vi "eventp.vi"() -> ()   [LabVIEW 2020]
panel:
  out "error out 2":errorcluster
  out "refnum out 2":refnum<file>
  in  "Write":bool
  out "refnum out":refnum<file>
  out "error out":errorcluster
  in  "Close File":bool
  in  "Path":path=path "C:/Users/rsKite/Documents/FSR DATA"
  out "File Name":string
  in  "Weight":string
  in  "Trial":string caption="Participant Name (FirstLast)"
  in  "Create/OpenFile":bool
  in  "OK Button":bool
  in  "stop":bool
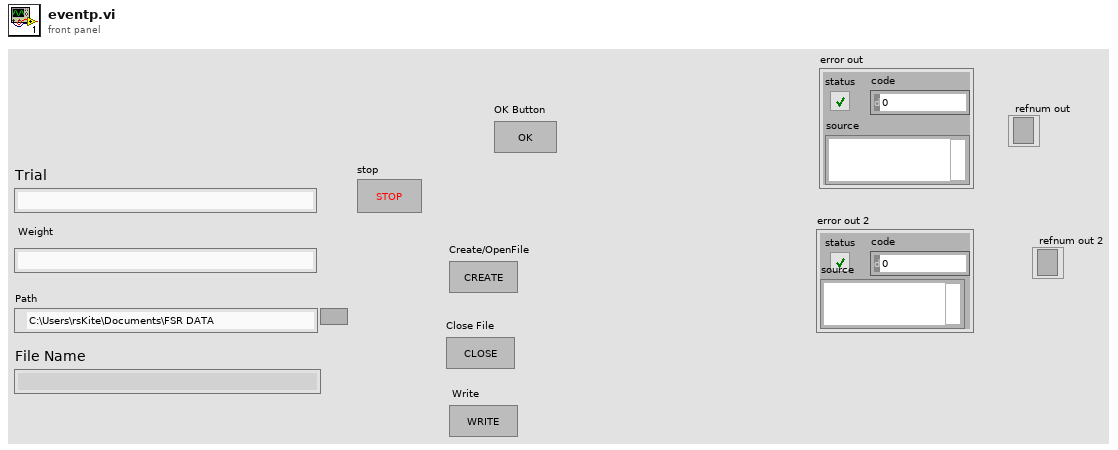
[diagram p1: front panel]
types:
  T1 = enum16{"open", "replace", "create", "open or create", "replace or create", "replace or create with confirmation"}
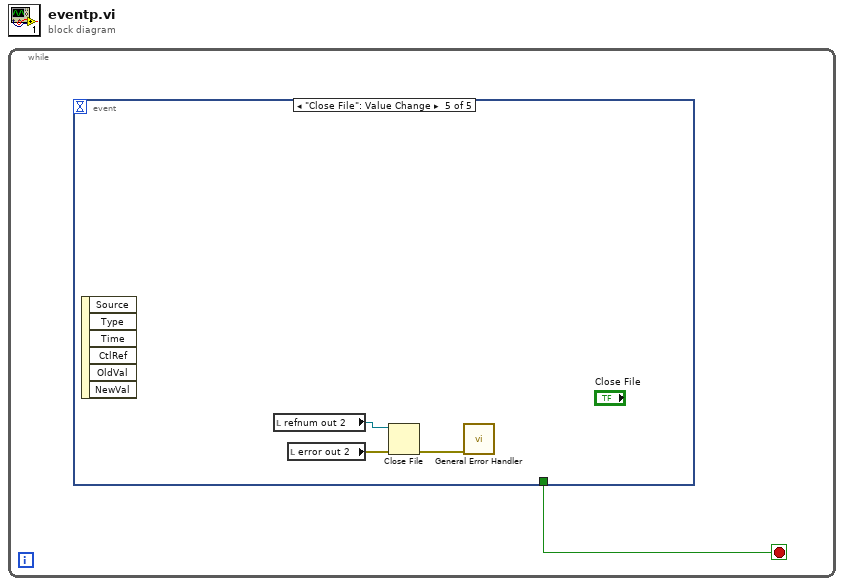
[diagram p0: block diagram]
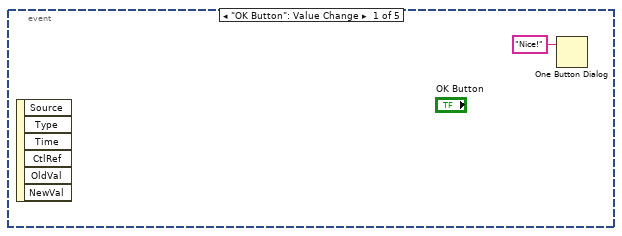
[diagram p2: hidden frame]
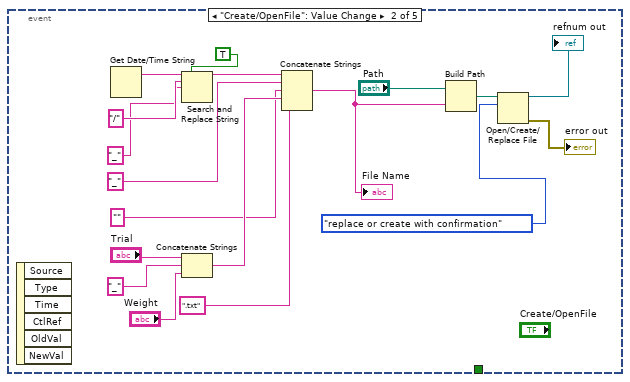
[diagram p3: hidden frame]
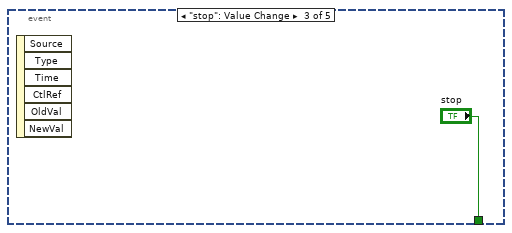
[diagram p4: hidden frame]
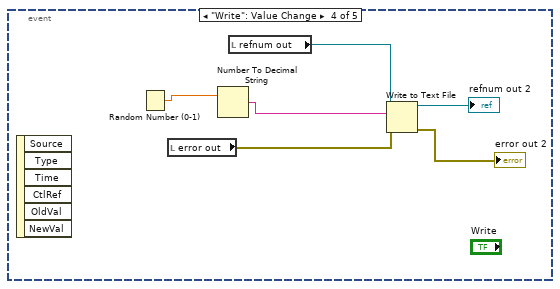
[diagram p5: hidden frame]
diagram:
  n1 = while {
    stop <- w1 stop-if-true
    n2 = event shown="[4] \"Close File\": Value Change" {
      selector: _ -> [_ _ _ _ _]
      dyn-events: _ -> [_ _ _ _ _]
      timeout: _ -> [_ _ _ _ _]
      tunnel: [_ _ "stop" _ _] -> w1
      event "OK Button": Value Change {
        n3 = event-data() -> ()  [unwired: 1 in, 6 out]
        n4 = One Button Dialog(message="Nice!") -> ()  [unwired: 1 in, 1 out]
      }
      event "Create/OpenFile": Value Change {
        n5 = event-data() -> ()  [unwired: 1 in, 6 out]
        n6 = Get Date/Time String() -> (date string=w16:string)  [unwired: 3 in, 1 out]
        n7 = Search and Replace String(replace all?=TRUE ("replace all? (F)"), input string=w16, search string="/", replace string="_" ("replace string (\"\")")) -> (result string=w18:string)  [unwired: 4 in, 3 out]
        n8 = Concatenate Strings("Trial", "_" ("string"), "Weight") -> (w17:string)
        n9 = Concatenate Strings(w18, "_" ("string"), "" ("string"), w17, ".txt" ("string")) -> (w8:string)
        "File Name" <- w8
        n10 = Build Path(base path="Path", name or relative path=w8) -> (appended path=w6:path)
        n11 = Open/Create/Replace File(file path (use dialog)=w6, operation (0:open)=T1."replace or create with confirmation") -> (refnum out=→"refnum out":refnum<file>, error out=→"error out":errorcluster)  [unwired: 4 in, 1 out]
      }
      event "stop": Value Change {
        n12 = event-data() -> ()  [unwired: 1 in, 6 out]
      }
      event "Write": Value Change {
        n13 = event-data() -> ()  [unwired: 1 in, 6 out]
        n14 = Random Number (0-1)() -> (number: 0 to 1=w25:dbl)
        n15 = local read "error out"() -> (w26:errorcluster)
        n16 = Number To Decimal String(number=w25) -> (decimal integer string=w24:string)  [unwired: 1 in]
        n17 = local read "refnum out"() -> (w27:refnum<file>)
        n18 = Write to Text File(file (use dialog)=w27, text=w24, error in=w26) -> (refnum out=→"refnum out 2":refnum<file>, error out=→"error out 2":errorcluster)  [unwired: 1 in, 1 out]
      }
      event "Close File": Value Change {
        n19 = event-data() -> ()  [unwired: 1 in, 6 out]
        n20 = local read "refnum out 2"() -> (w28:refnum<file>)
        n21 = local read "error out 2"() -> (w29:errorcluster)
        n22 = Close File(refnum=w28, error in=w29) -> (error out=w30:errorcluster)  [unwired: 1 out]
        n23 = call <vilib>:"General Error Handler.vi"("error in (no error)"=w30) -> ()  [unwired: 10 in, 5 out]
      }
    }
  }
